vi "geophys.vi"() -> ()   [LabVIEW 2018]
doc: "I. Description:\nThis example demonstrates how to continuously acquire and generate data at the same time, synchronized with one another.\n\nII. Instructions for Running:\n1. Select the physical channel to correspond to where your signal is input on the DAQ device. Also, select the corresponding channel for where your signal is being generated.\n2. Enter the minimum and maximum voltage ranges.\nNote: For better accuracy try to match the input range to the expected voltage level of the measured signal.\n3. Set the sample rate of the acquisition.\nNote: The rate should be at least twice as fast as the maximum frequency component of the signal being acquired. \n6. Select the Rate for the generation\n7. Select what type of signal to generate and the amplitude.\nNote: This example requires two DMA channels to run. If your hardware does not support two DMA channels, you need to set the Data Transfer Mechanism property for the Analog Output Task to use \"Interrupts\". The Data Transfer Mechanism property is located in the DAQmx Channel Property hierarchy at:\n\nDAQmx Channel Property Node>>Analog Output>>General Properties>>Advanced>>Data Transfer and Memory>>Data Transfer Mechanism\n\nRefer to your device documentation to determine how many DMA channels are supported for your hardware.\n\nIII. Block Diagram Steps:\n1. Create an analog input voltage channel. Also, create an analog output voltage channel.\n2. Set the rate for the sample clock. Additionally, define the sample mode to be continuous. Also, set the sample clock rate for the signal generation.\n2a. Call the Get Terminal Name with Device Prefix VI. This will take a Task and a terminal and create a properly formatted device + terminal name to use as the source of the Trigger.\n3. Define the parameters for a Digital Edge Start Trigger. Set the Analog output to trigger off the AI Start Trigger. This is an internal trigger signal.\n4. Use the Basic Function Generator VI to create the signal to be generated.\n5. Call the Start VI to arm the two functions. Make sure the analog output is armed before the analog input. This will ensure both will start at the same time.\n6. Read the waveform data in a loop until the user hits the stop button or an error occurs. The Is Task Done? VI is used to check for errors in the Analog Output Task.\n7. Call the Clear VI to Clear the Task\n8. Use the popup dialog box to display an error if any.\n\nIV. I/O Connections Overview:\nMake sure your signal input/output terminals match the Physical Channel I/O controls."
panel:
  in  "Périphérique":tag="Dev1"
  in  "Nombre d'échantillons (Par entrée)":i32=5000
  in  "Fréquence d'acquisition (échantillons/s)":dbl=2500.0
  out "data":dynamicdata(graph) caption="Données"
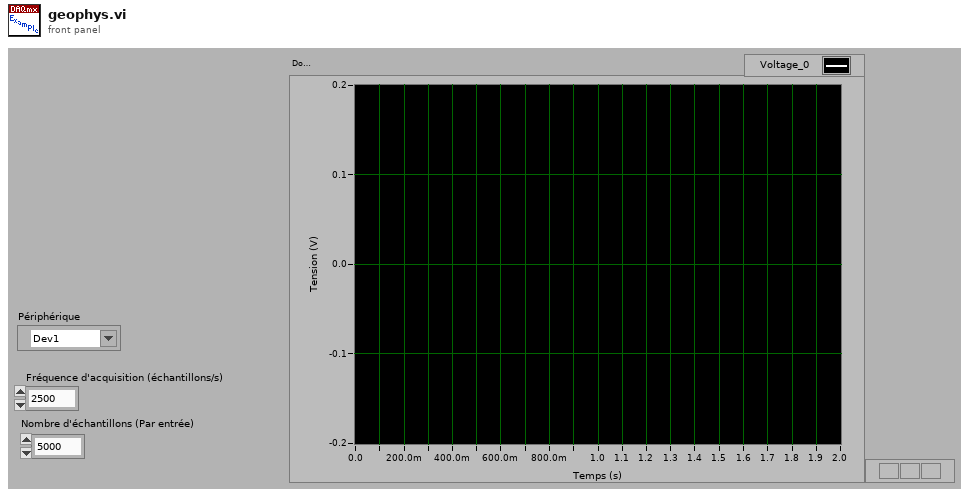
[diagram p1: front panel]
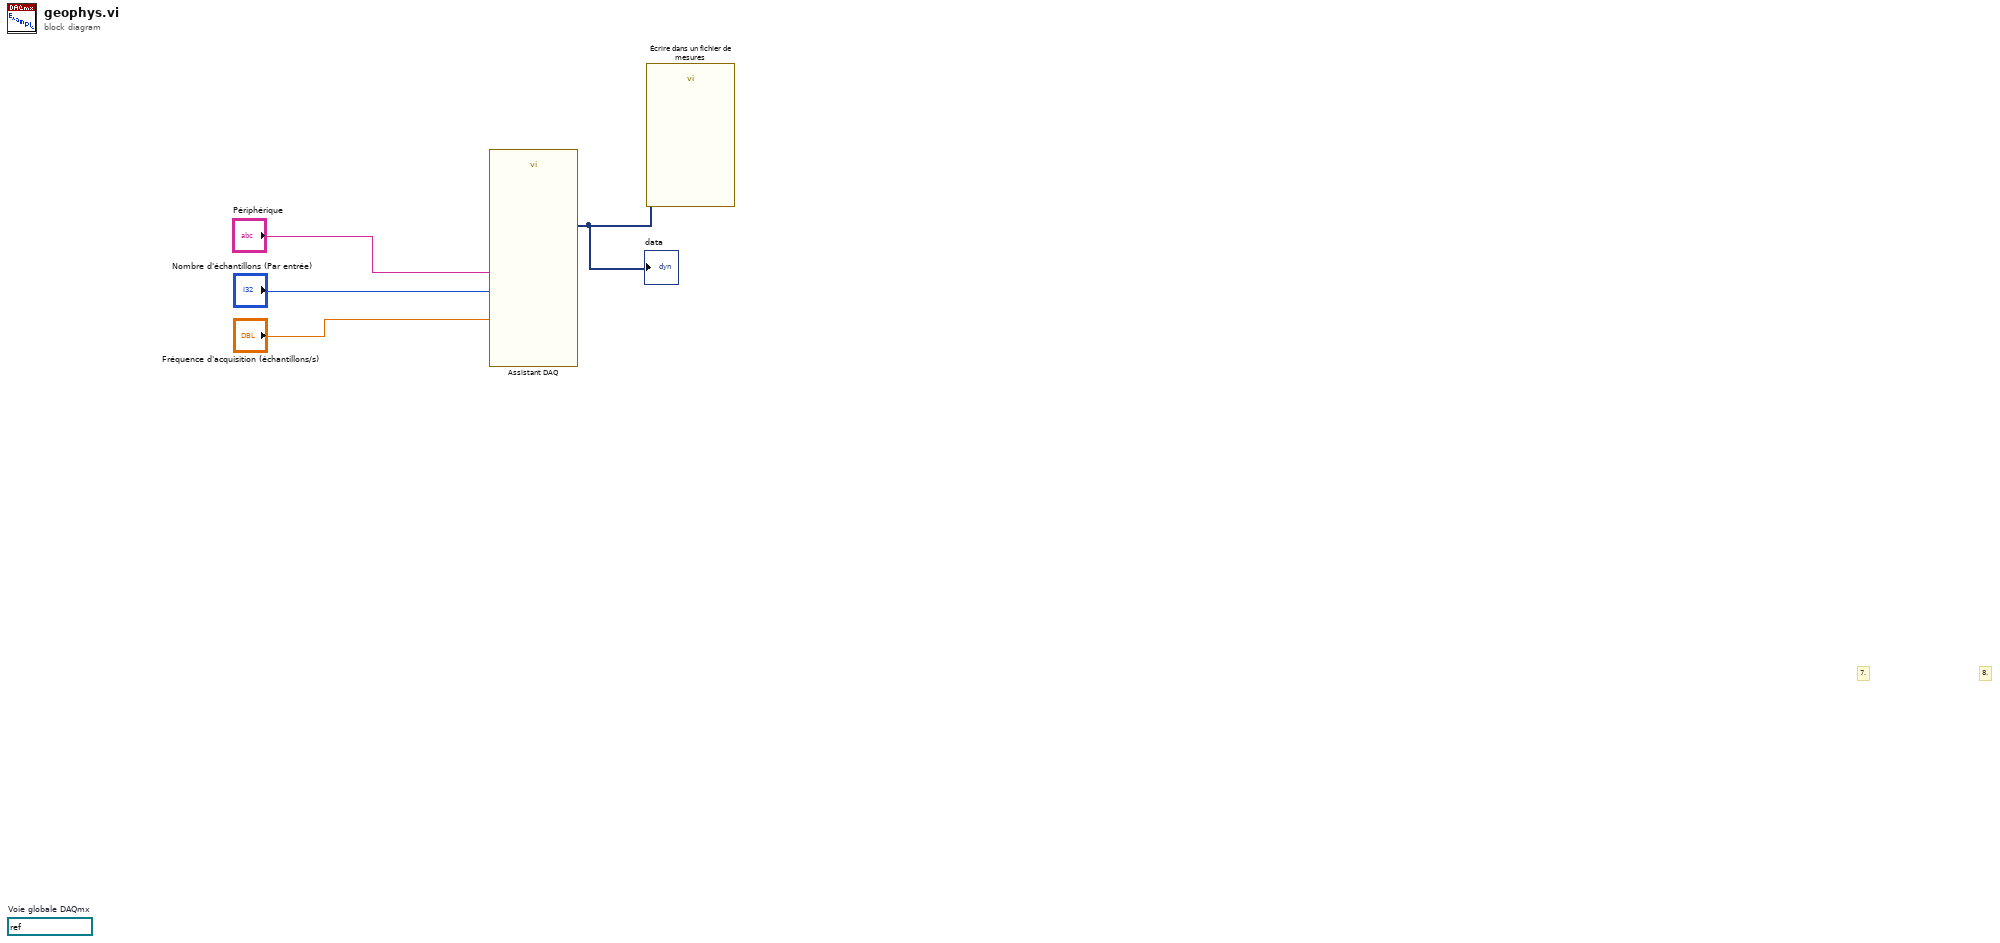
[diagram p0: block diagram]
diagram:
  (unwired) refnum<k21> "dTriggerP13"  # Voie globale DAQmx
  # "8."
  # "7."
  n1 = call "Assistant DAQ"("rate"="Fréquence d'acquisition (échantillons/s)", "number of samples"="Nombre d'échantillons (Par entrée)", "device name"="Périphérique") -> ("data"=w4:dynamicdata)  [unwired: 14 in, 2 out]
  "data" <- w4
  n2 = call "Écrire dans un fichier de mesures"("Signals"=w4) -> ()  [unwired: 16 in, 3 out]
